vi "pigeon_ver4_1.vi"() -> ()   [LabVIEW 2017]
uses:
  <vilib>/Platform/TimedLoop/XDataNode/timing_clust.ctl
  <vilib>/Platform/TimedLoop/XDataNode/nitl_modes.ctl
  <vilib>/Platform/TimedLoop/XDataNode/wakeup.ctl
  <vilib>/rvi/Emulation/niFpgaGetClockAttributes.vi
  <vilib>/rvi/Emulation/niFpgaSctlEmulationGetInTimedLoop.vi
  <vilib>/rvi/Emulation/niFpgaEmulationReportErrorSimple.vi
  <vilib>/rvi/eio/common/nirviEmuTemplateMethod_errors.vi
  <vilib>/rvi/Emulation/niFpgaProcessEmulError.vi
  <vilib>/rvi/Emulation/niFpgaCriticalErrorInLSC.vi
  <vilib>/rvi/occurrence/nirviWaitOnOccurrenceBase.vi
  <vilib>/rvi/Memory/Memory_Emulation/nirvimemoryFastEmulation.vi
  <vilib>/rvi/Memory/Memory_Emulation/nirvimemoryEmulation.vi
  <vilib>/rvi/Emulation/niFpgaEmulationIsFPGAContextNoSignature.vi
  <vilib>/rvi/DataTransferAndStorage/Container/Common/niFpgaContainerGetUniqueNameForEmu.vi
  <vilib>/rvi/errors/nirviReportUnexpectedCaseInternalError (U32).vi
  <vilib>/rvi/interface/RandomDataEmulation/niFpgaRandomDataHandleErrors.vi
  <vilib>/eio/EIONode/EIONode.xnode
  <vilib>/Platform/TimedLoop/XDataNode/XDataNode.xnode
  <vilib>/rvi/DataTransferAndStorage/Container/XNode/niFpgaContainer.xnode
  <vilib>/rvi/interface/RandomDataEmulation/nirviRandomDataFpgaReadWriteTemplate.vi
  <vilib>/Platform/TimedLoop/XDataNode/XDNodeRunTimeDep.lvlib
panel:
  out "It 2":fxp<+,32,8>
  out "ramp ctr 2":i32
  in  "AO0 2":i16
  out "It":fxp<+,32,8>
  out "ramp ctr":i32
  out "Numeric":i16
  in  "analog ramp on":bool
  out "AI2":i16
  in  "Tab Control":enum32{"pigeon"}(tab)
  in  "Digital Reset":bool
  in  "Emergency Stop":bool
  in  "AO0_pigeon":i16
  in  "AO7":i16
  in  "AO6":i16
  out "trigger AI1":bool
  in  "Tab Control 2":T1(tab)
  out "head ip":u16
  out "nxt ip output":u16
  out "forctr output":u16
  out "curr ip":u16
  out "for ctr":u16
  out "for N":u16
  in  "square wave  on?":bool
  in  "square wave period":i32
  in  "IGBTswitch":bool caption="IGBT Switch circular"
  in  "Manual Override":bool
  in  "circular coil current":i16(slide) scale=0.0..32768.0
  in  "analog ramp period":i16
  in  "analog ramp on  2":bool
  in  "End Current":fxp<+,16,16>
  out "circ coil ramp loop end?":bool=TRUE
  out "ramp start val":fxp<+,15,15>
  out "cooling intensity start val":fxp<+,15,15>
  in  "End Cooling Intensity":fxp<+,16,16>
  in  "cooling intensity ramp on":bool
  out "cooling power ramp loop end?":bool=TRUE
  in  "ramp time [10*us]":fxp<+,16,16>
  out "delta cooling power /dT":fxp<+/-,32,9>
  in  "cooling ramp time [10*us]":fxp<+,16,16>
  out "deltaI/T":fxp<+/-,32,9>
  out "PD1":i16
  out "PD2":i16
  out "PD3":i16
  out "FIFO size":i16
  in  "AO0":i16
  in  "AO1":i16
  in  "AO2":i16
  in  "Run program":bool
  in  "halt processor":bool
  out "control flags":i8 format="%b"
  in  "host operation":i16
  in  "address":u16
  in  "data1":u16
  in  "data2":i32
  in  "repeat program":i32
  out "IP address":i16
  out "PMT1":i16=-4740
  out "ReA":i32
  out "RegB":i16
  out "RegC":i16
  out "exttrigger":bool=TRUE
  out "AI1":i16=161
  out "RegD":i16
  in  "AO4":i16
  in  "AO3":i16
  out "Connector0/AI0":i16
  in  "AO5":i16
  in  "AO5_pigeon":i16
  out "connector 0 DIO":bool[](array[boolean])
  out "connector 1 DIO":bool[](array[boolean])
  out "connector 2 DIO":bool[](array[boolean])
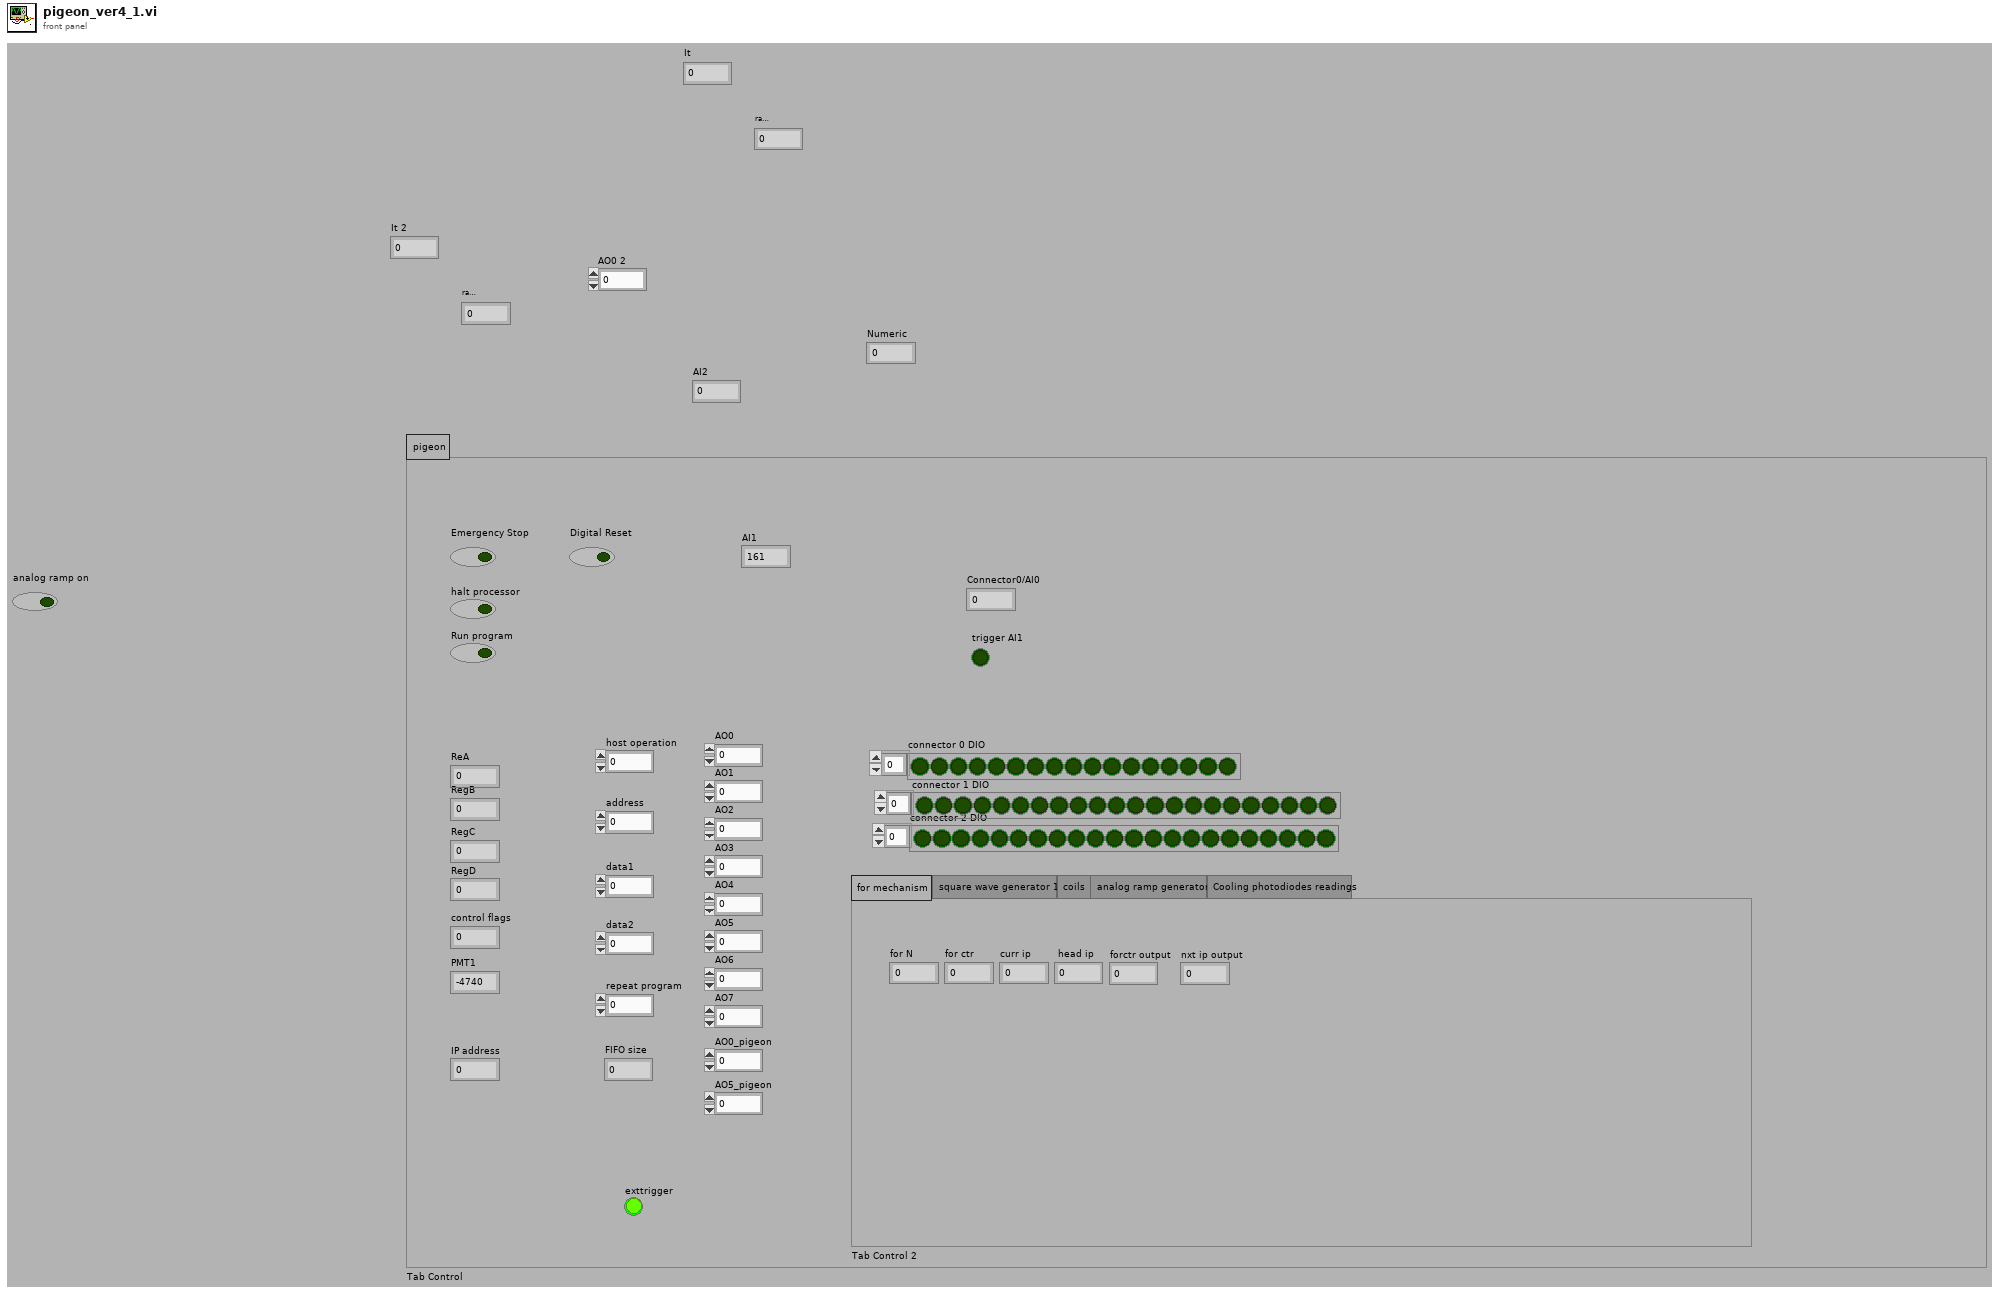
[diagram p1: front panel]
types:
  T1 = enum32{"for mechanism", "square wave generator 1", "coils", "analog ramp generator", "Cooling photodiodes readings"}
  T2 = typedef "XDNodeRunTimeDep.lvlib/timing_clust.ctl" = cluster{"Expected End [f-1]":u64, "Actual End [f-1]":u64, "Finished Late? [f-1]":bool, "Expected End [i-1]":u64, "Actual End [i-1]":u64, "Finished Late? [i-1]":bool, "Expected Start [i]":u64, "Actual Start [i]":u64, "Expected Start [f]":u64, "Actual Start [f]":u64, "Source Name":string, "Structure Name":string, "Period":i64, "Deadline":i64, "Offset":i64, "Start":i64, "Priority":i32, "Timeout":i32, "Mode":T3, "Wakeup Reason":T4, "Error":errorcluster, "Source Type":string, "Secondary Source Type":string, "Global End Time":u64, "Global Start Time":u64, "Frame Duration":u64, "Iteration Duration":u64, "Assigned CPU":i32, "I/O Scan Engine Mode":u32}
  T3 = typedef "XDNodeRunTimeDep.lvlib/nitl_modes.ctl" = enum32{"No Change", "Process missed periods, maintain original phase", "Discard missed periods, maintain original phase", "Process missed periods, ignore original phase", "Discard missed periods, ignore original phase"}
  T4 = typedef "XDNodeRunTimeDep.lvlib/wakeup.ctl" = enum32{"Normal", "Aborted", "Asynchronous wakeup", "Timing source error", "Timed loop error", "Timeout"}
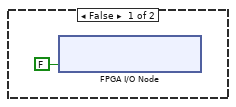
[diagram p2: hidden frame]
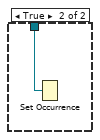
[diagram p3: hidden frame]
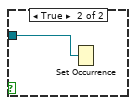
[diagram p5: hidden frame]
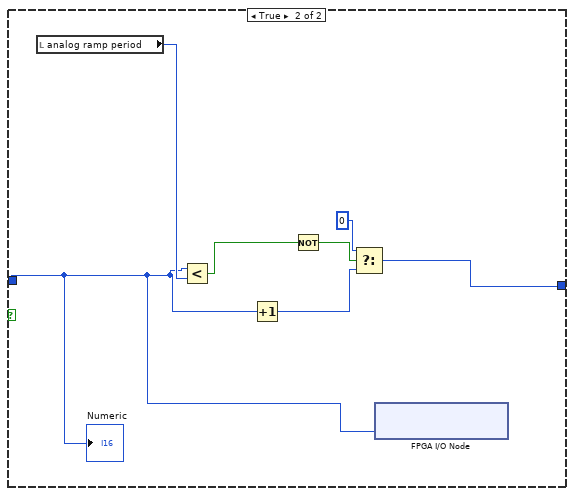
[diagram p6: hidden frame]
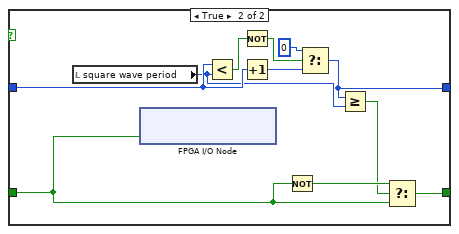
[diagram p7: hidden frame]
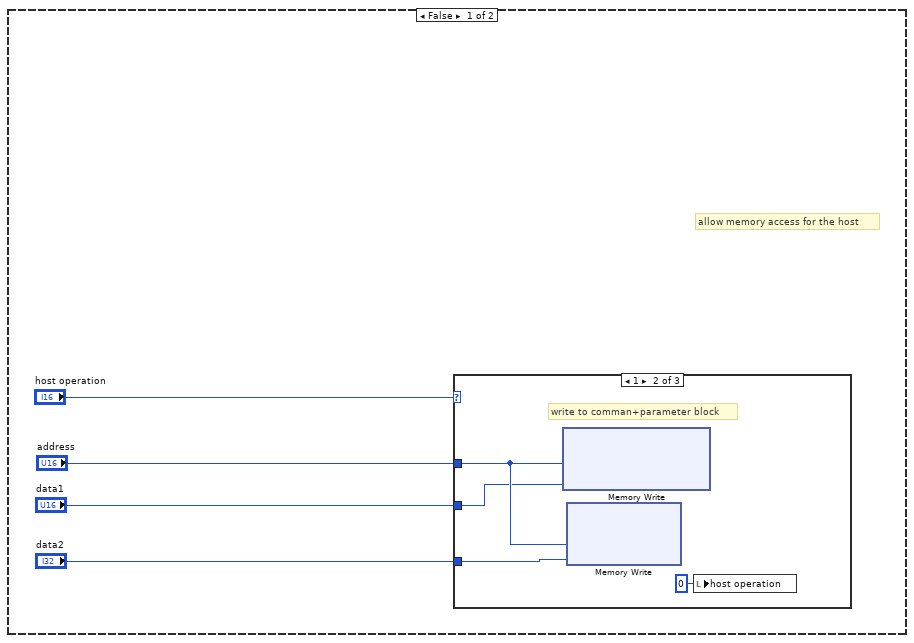
[diagram p8: hidden frame]
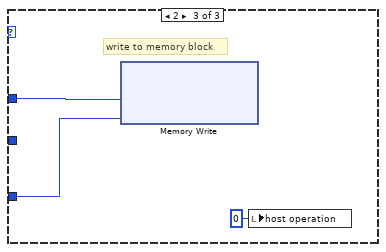
[diagram p10: hidden frame]
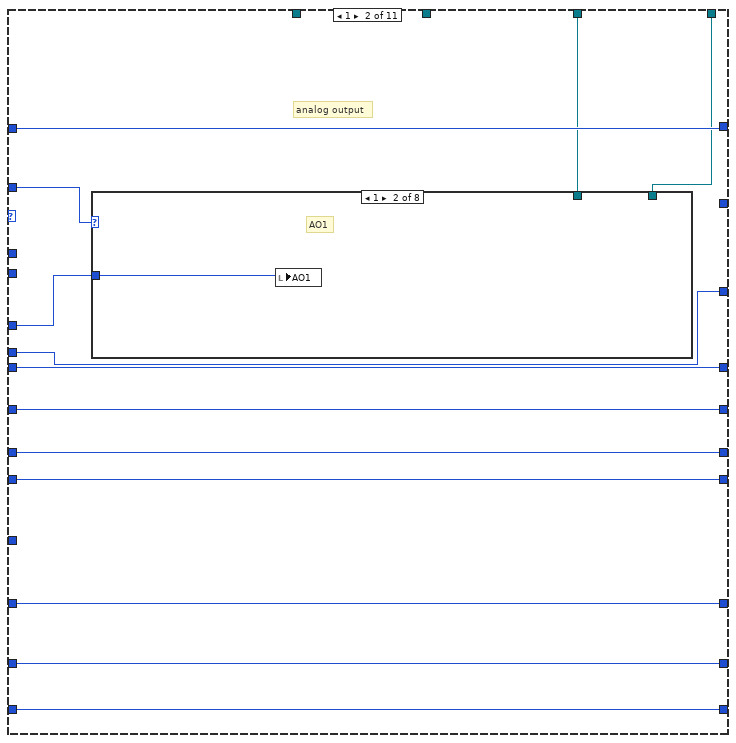
[diagram p12: hidden frame]
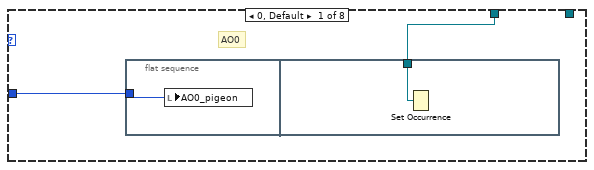
[diagram p13: hidden frame]
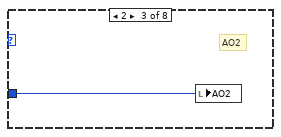
[diagram p14: hidden frame]
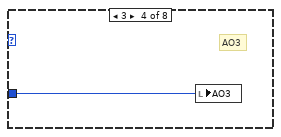
[diagram p15: hidden frame]
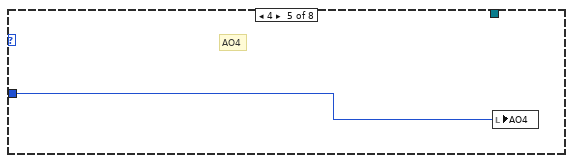
[diagram p16: hidden frame]
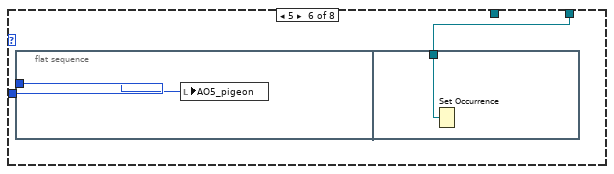
[diagram p17: hidden frame]
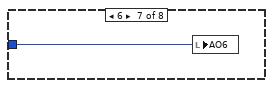
[diagram p18: hidden frame]
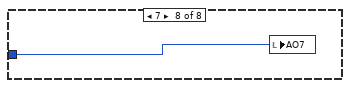
[diagram p19: hidden frame]
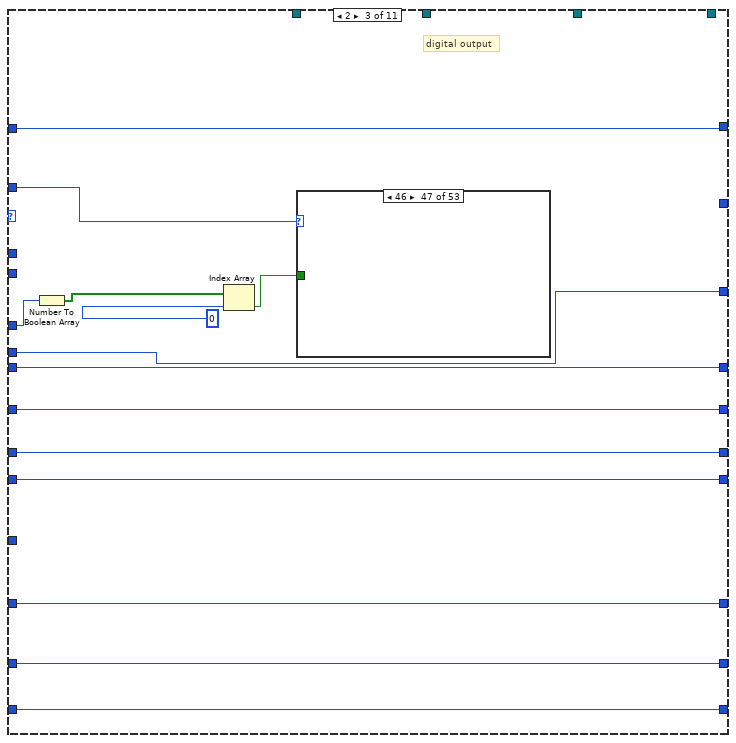
[diagram p20: hidden frame]
diagram:
  w13 = refnum<k21> "40 MHz Onboard Clock" ("FPGA Clock")
  # "circular coil analog ramp occurance"
  # "analog ramp generator"
  # "Analog read block for loading time"
  # "Square Wave Generator Block\nonly Connector1/DIO6 now supports this"
  # "RegB: accumulates flag[0] (results of if condition) to see how many bright events occured\nRegC: loop counter (for GenRepeatSeq)\nRegA: (sub) loop counter (for Gen Wait), #of     photons \nRegB:counter"
  # "flags[0]:result of the if statement\nflags[1]:reset photon counters\nflags[2]:count FIFO size\nflag3[3]:exttrigger\nflag4[4]:trigger MOT fluoresence counter\nflags[7]:halt and exit program"
  # "Digital pin layout\n----------------------------------------------------------------\n\n-----Connector0-----\nC0DIO0-8  -> Rack DIO 0-8\n\n-----Connector2-----\nC2DIO0  -> Rack DI9 external trigger \nC2DIO1-4  -> Rack DIO 10-13\nC2DIO5 -> integrator hold (single BNC)\nC2DIO6-10 D\\A voltage output\nC2DIO22-23 PMTs\nC2DIO32-39 stepmotors control"
  # "analog pin layout\n---------------------------------------------------------------\n\n------connector0-----\nAO0 VCO 422\nAO1 VCO 1092\nAO2 VCO optical pumping\nAO3 408 DC current control\nAO4 422 intensitiy mixer\nAO5 (used to be endcap N) B field feedforward\nAO6 endcap S\nAO7 674 intensity setpoint controller\n\nAI0 B field feed forward"
  n1 = case shown="False" "Digital Reset" {
    frame False {
    }
    frame True {
    }
  }
  n2 = Generate Occurrence() -> (w2:refnum<k4>)
  n3 = while {
    tunnel: w2 -> [w16]
    stop <- FALSE stop-if-true
    n4 = flat-sequence {
      tunnel: w16 -> [w18]
      frame #0 {
        n5 = Wait on Occurrence(2:w18) -> ()  [unwired: 2 in, 1 out]
      }
      frame #1 {
        # "delta I/T"
        n6 = local read "AO5"() -> (w20:i16)
        n7 = To Fixed-Point(number=w20) -> (fixed-point=w19:fxp<+,15,15>)  [unwired: 1 in]
        "cooling intensity start val" <- w19
        n8 = Subtract(x="End Cooling Intensity", y=w19) -> (x-y=w29:fxp<+/-,16,16>)
        n9 = Multiply(x="cooling ramp time [10*us]", y=fxp<+,16,16> 10.0) -> (x*y=w27:fxp<+,32,32>)
        n10 = Divide(x=w29, y=w27) -> (x/y=w28:fxp<+/-,32,16>)
        "delta cooling power /dT" <- w28
        n11 = while {
          tunnel: w28 -> [w41]
          tunnel: w19 -> [w40]
          tunnel: w29 -> [w39]
          tunnel: "End Cooling Intensity" -> [w38]
          shift-right: [w33] -> _
          shift-left: i16 0 -> [w34]
          tunnel: [w31] -> w22
          tunnel: [w30] -> w21
          stop <- w30 stop-if-true
          n12 = flat-sequence {
            tunnel: w38 -> [w44]
            tunnel: w39 -> [w45]
            tunnel: [w45] -> w37
            tunnel: [w44] -> w36
            tunnel: [w43] -> w35
            tunnel: w34 -> [w43]
            tunnel: [w42] -> w32
            tunnel: [w61] -> w30
            tunnel: w41 -> [w60]
            tunnel: w40 -> [w59]
            tunnel: w37 -> [w58]
            tunnel: w36 -> [w57]
            tunnel: w35 -> [w50]
            tunnel: [w51] -> w33
            tunnel: w32 -> [w49]
            tunnel: [w46] -> w31
            frame #0 {
              w42 = u32 2 ("Count(uSec)")
              n13 = call "Loop Timer2"("Count(uSec)"=w42) -> ()  [unwired: 1 out]
            }
            frame #1 {
              # "elapsed time"
              n14 = Multiply(x=w49, y=w50) -> (x*y=w48:fxp<+,15,15>)
              n15 = Increment(x=w50) -> (x+1=w51:i32)
              "ramp ctr 2" <- w51
              n16 = Greater?(x=w58, y=fxp<+/-,31,9> 0.0) -> (0:w54:bool)
              n17 = Multiply(x=w60, y=w48) -> (x*y=w56:fxp<+/-,32,16>)
              n18 = Add(x=w59, y=w56) -> (x+y=w46:fxp<+,15,15>)
              "It 2" <- w46
              n19 = To Word Integer(number=w46) -> (16bit integer=w47:i16)
              n20 = Greater?(x=w46, y=w57) -> (0:w53:bool)
              n21 = Not(x=w53) -> (.not. x?=w52:bool)
              n22 = local write "AO5"(w47) -> ()
              n23 = Select(t=w53, s=w54, f=w52) -> (s? t:f=w61:bool)
            }
          }
        }
        "cooling power ramp loop end?" <- w21
        n24 = local write "cooling intensity start val"(w22) -> ()
      }
    }
  }
  n25 = while {
    tunnel: w2 -> [w63]
    stop <- FALSE stop-if-true
    n26 = case shown="False" "cooling intensity ramp on" {
      tunnel: w63 -> [_ w65]
      frame False {
      }
      frame True {
        n27 = Set Occurrence(w65) -> ()
      }
    }
  }
  n28 = while "Analog out loop" {
    stop <- FALSE stop-if-true
    n29 = Select(t=i16 16385, s="IGBTswitch", f=i16 0) -> (s? t:f=w74:i16)
    n30 = Select(t="circular coil current", s="Manual Override", f="AO0") -> (s? t:f=w68:i16)
    n31 = Select(t=w74, s="Manual Override", f="AO3") -> (s? t:f=w73:i16)
    n32 = xnode "FPGA I/O Node"("Connector0/AO0"=w68, "Connector0/AO1"="AO1", "Connector0/AO2"="AO2", "Connector0/AO3"=w73, "Connector0/AO4"="AO4", "Connector0/AO5"="AO5", "Connector0/AO6"="AO6", "Connector0/AO7"="AO7") -> ("Connector0/AI1"=→"AI1":i16, "Connector0/AI2"=→"AI2":i16)  [unwired: 10 in, 10 out]
  }
  n33 = node-c288(w13) -> (w15:T2)
  n34 = timed-loop {
    timing: w15 -> [_]
    timing-out: [_] -> w14
    shift-right: [w98] -> _
    shift-left: _ -> [w87]
    shift-right: [w91] -> _
    shift-left: _ -> [w100]
    shift-right: [w93] -> _
    shift-left: _ -> [w94]
    stop <- FALSE stop-if-true
    (unwired) FALSE
    n35 = local read "control flags"() -> (w95:i8)
    n36 = xnode "FPGA I/O Node"() -> ("Connector2/DIO0"=→"exttrigger":bool)  [unwired: 1 in, 1 out]
    n37 = xnode "FPGA I/O Node"() -> ("Connector0/DIO0"=w91:bool)  [unwired: 1 in, 1 out]
    n38 = Number To Boolean Array(number=w95) -> (Boolean array=w96:bool[])
    n39 = Increment(x=w87) -> (x+1=w88:u16)
    n40 = Index Array(array=w96, index=1) -> (element=w93:bool)
    n41 = Greater?(x=w91, y=w100) -> (0:w90:bool)
    n42 = Not Equal?(x=w93, y=w94) -> (x != y?=w85:bool)
    n43 = Select(t=w88, s=w90, f=w87) -> (s? t:f=w99:u16)
    n44 = Select(t=u16 0, s=w85, f=w99) -> (s? t:f=w98:u16)
    "PMT1" <- w98
  }
  n45 = Generate Occurrence() -> (w6:refnum<k4>)
  n46 = local write "cooling power ramp loop end?"(FALSE ("ramp loop end?")) -> ()
  n47 = local write "circ coil ramp loop end?"(FALSE ("ramp loop end?")) -> ()
  n48 = node-c288(w14) -> ()
  n49 = while {
    tunnel: w6 -> [w104]
    stop <- FALSE stop-if-true
    n50 = case shown="False" "analog ramp on  2" {
      tunnel: w104 -> [_ w106]
      frame False {
      }
      frame True {
        n51 = Set Occurrence(w106) -> ()
      }
    }
  }
  n52 = while {
    tunnel: w6 -> [w107]
    stop <- FALSE stop-if-true
    n53 = flat-sequence {
      tunnel: w107 -> [w109]
      frame #0 {
        n54 = Wait on Occurrence(2:w109) -> ()  [unwired: 2 in, 1 out]
      }
      frame #1 {
        # "delta I/T"
        n55 = local read "AO0"() -> (w114:i16)
        "ramp start val" <- w114
        n56 = Divide(x=fxp<+,15,15> 220.0, y=i16 32767) -> (x/y=w115:fxp<+,32,16>)
        n57 = Multiply(x=w115, y=w114) -> (x*y=w113:fxp<+/-,48,32>)
        n58 = Subtract(x="End Current", y=w113) -> (x-y=w125:fxp<+/-,32,9>)
        n59 = Multiply(x="ramp time [10*us]", y=fxp<+,16,16> 10.0) -> (x*y=w123:fxp<+,32,32>)
        n60 = Divide(x=w125, y=w123) -> (x/y=w124:fxp<+/-,32,9>)
        "deltaI/T" <- w124
        n61 = Divide(x=fxp<+,15,15> 32767.0, y=fxp<+,6,8> 220.0) -> (x/y=w126:fxp<+,15,15>)
        n62 = while {
          tunnel: w126 -> [w140]
          tunnel: w124 -> [w139]
          tunnel: w113 -> [w138]
          tunnel: w125 -> [w137]
          tunnel: "End Current" -> [w136]
          shift-right: [w130] -> _
          shift-left: i16 0 -> [w131]
          tunnel: [w128] -> w111
          tunnel: [w127] -> w110
          stop <- w127 stop-if-true
          n63 = flat-sequence {
            tunnel: w136 -> [w143]
            tunnel: w137 -> [w144]
            tunnel: w140 -> [w145]
            tunnel: [w145] -> w135
            tunnel: [w144] -> w134
            tunnel: [w143] -> w133
            tunnel: [w142] -> w132
            tunnel: w131 -> [w142]
            tunnel: [w141] -> w129
            tunnel: [w161] -> w127
            tunnel: w139 -> [w160]
            tunnel: w138 -> [w159]
            tunnel: w135 -> [w162]
            tunnel: w134 -> [w158]
            tunnel: w133 -> [w157]
            tunnel: w132 -> [w149]
            tunnel: [w150] -> w130
            tunnel: w129 -> [w148]
            tunnel: [w146] -> w128
            frame #0 {
              w141 = u32 2 ("Count(uSec)")
              n64 = call "Loop Timer"("Count(uSec)"=w141) -> ()  [unwired: 1 out]
            }
            frame #1 {
              # "elapsed time"
              n65 = Multiply(x=w148, y=w149) -> (x*y=w147:u32)
              n66 = Increment(x=w149) -> (x+1=w150:i32)
              "ramp ctr" <- w150
              n67 = Greater?(x=w158, y=fxp<+/-,31,9> 0.0) -> (0:w154:bool)
              n68 = Multiply(x=w160, y=w147) -> (x*y=w156:fxp<+/-,32,9>)
              n69 = Add(x=w159, y=w156) -> (x+y=w153:fxp<+,32,8>)
              "It" <- w153
              n70 = Multiply(x=w162, y=w153) -> (x*y=w146:i16)
              n71 = Greater?(x=w153, y=w157) -> (0:w152:bool)
              n72 = local write "AO0"(w146) -> ()
              n73 = Not(x=w152) -> (.not. x?=w151:bool)
              n74 = Select(t=w152, s=w154, f=w151) -> (s? t:f=w161:bool)
            }
          }
        }
        "circ coil ramp loop end?" <- w110
        n75 = local write "ramp start val"(w111) -> ()
      }
    }
  }
  n76 = while {
    shift-right: [w163] -> _
    shift-left: _ -> [w165]
    stop <- FALSE stop-if-true
    # "write Pulse to conn2/Dio26 on low->high transition of dio12. used for the trigger channel (channel 3) of the time tagger"
    n77 = xnode "FPGA I/O Node"() -> ("Connector2/DIO12"=w166:bool)  [unwired: 1 in, 1 out]
    n78 = Not(x=w165) -> (.not. x?=w164:bool)
    n79 = feedback-in #1(w166) -> ()
    n80 = feedback #1() -> (w163:bool)  [unwired: 1 in]
    n81 = case shown="True" w163 {
      frame False {
        n82 = xnode "FPGA I/O Node"("Connector2/DIO26"=FALSE) -> ()  [unwired: 1 in, 1 out]
      }
      frame True {
        n83 = call "Wait"("Count(uSec)"=u32 1) -> ()  [unwired: 1 out]
        n84 = xnode "FPGA I/O Node"("Connector2/DIO26"=TRUE) -> ()  [unwired: 1 in, 1 out]
      }
    }
    n85 = And(x=w164, y=w163) -> ()  [unwired: 1 out]
  }
  n86 = while {
    stop <- FALSE stop-if-true
    n87 = xnode "FPGA I/O Node"() -> ("Connector0/AI1"=→"PD1":i16, "Connector0/AI2"=→"PD2":i16, "Connector0/AI3"=→"PD3":i16)  [unwired: 3 in, 3 out]
  }
  n88 = Generate Occurrence() -> (w5:refnum<k4>)
  n89 = while {
    tunnel: w5 -> [w176]
    stop <- FALSE stop-if-true
    n90 = flat-sequence {
      tunnel: w176 -> [w177]
      frame #0 {
        n91 = Wait on Occurrence(2:w177) -> ()  [unwired: 2 in, 1 out]
      }
      frame #1 {
        n92 = local read "AO0_pigeon"() -> (w178:i16)
        n93 = local write "AO0"(w178) -> ()
      }
    }
  }
  n94 = while {
    stop <- FALSE stop-if-true
    n95 = xnode "FPGA I/O Node"() -> ("Connector0/DIO0"=w241:bool, "Connector0/DIO1"=w240:bool, "Connector0/DIO2"=w239:bool, "Connector0/DIO3"=w238:bool, "Connector0/DIO4"=w237:bool, "Connector0/DIO5"=w236:bool, "Connector0/DIO6"=w235:bool, "Connector0/DIO7"=w234:bool, "Connector0/DIO8"=w233:bool, "Connector0/DIO9"=w232:bool, "Connector0/DIO10"=w231:bool, "Connector0/DIO11"=w230:bool, "Connector0/DIO12"=w229:bool, "Connector0/DIO13"=w228:bool, "Connector0/DIO14"=w227:bool, "Connector0/DIO15"=w226:bool)  [unwired: 16 in, 16 out]
    n96 = Build Array(w241, w240, w239, w238, w238, w237, w236, w235, w234, w233, w232, w231, w230, w229, w228, w227, w226) -> (→"connector 0 DIO":bool[])
    n97 = xnode "FPGA I/O Node"() -> ("Connector1/DIO0"=w224:bool, "Connector1/DIO1"=w223:bool, "Connector1/DIO2"=w222:bool, "Connector1/DIO3"=w221:bool, "Connector1/DIO4"=w220:bool, "Connector1/DIO5"=w219:bool, "Connector1/DIO6"=w218:bool, "Connector1/DIO7"=w217:bool, "Connector1/DIO8"=w216:bool, "Connector1/DIO9"=w215:bool, "Connector1/DIO10"=w214:bool, "Connector1/DIO11"=w213:bool, "Connector1/DIO12"=w212:bool, "Connector1/DIO13"=w211:bool, "Connector1/DIO15"=w210:bool, "Connector1/DIO16"=w209:bool, "Connector1/DIO17"=w208:bool, "Connector1/DIO18"=w207:bool, "Connector1/DIO19"=w206:bool, "Connector1/DIO20"=w205:bool, "Connector1/DIO21"=w204:bool, "Connector1/DIO22"=w203:bool)  [unwired: 23 in, 24 out]
    n98 = Build Array(w224, w223, w222, w221, w220, w219, w218, w217, w216, w215, w214, w213, w212, w211, w210, w209, w208, w207, w206, w205, w204, w203) -> (→"connector 1 DIO":bool[])
    n99 = xnode "FPGA I/O Node"() -> ("Connector2/DIO0"=w201:bool, "Connector2/DIO1"=w200:bool, "Connector2/DIO2"=w199:bool, "Connector2/DIO3"=w198:bool, "Connector2/DIO4"=w197:bool, "Connector2/DIO5"=w196:bool, "Connector2/DIO6"=w195:bool, "Connector2/DIO7"=w194:bool, "Connector2/DIO8"=w193:bool, "Connector2/DIO9"=w192:bool, "Connector2/DIO10"=w191:bool, "Connector2/DIO11"=w190:bool, "Connector2/DIO12"=w189:bool, "Connector2/DIO12"=w188:bool, "Connector2/DIO14"=w187:bool, "Connector2/DIO15"=w186:bool, "Connector2/DIO16"=w185:bool, "Connector2/DIO17"=w184:bool, "Connector2/DIO18"=w183:bool, "Connector2/DIO19"=w182:bool, "Connector2/DIO20"=w181:bool, "Connector2/DIO21"=w180:bool)  [unwired: 23 in, 24 out]
    n100 = Build Array(w201, w200, w199, w198, w197, w196, w195, w194, w193, w192, w191, w190, w189, w188, w187, w186, w185, w184, w183, w182, w181, w180) -> (→"connector 2 DIO":bool[])
  }
  n101 = Generate Occurrence() -> (w3:refnum<k4>)
  n102 = while "main loop" {
    tunnel: w13 -> [w247]
    tunnel: w6 -> [w246]
    tunnel: w5 -> [w245]
    tunnel: w3 -> [w244]
    tunnel: w2 -> [w243]
    stop <- FALSE ("stop") stop-if-true
    n103 = case shown="True" "Run program" {
      tunnel: w247 -> [_ w265]
      tunnel: w246 -> [_ w264]
      tunnel: w245 -> [_ w263]
      tunnel: w244 -> [_ w262]
      tunnel: w243 -> [_ w261]
      frame False {
        # "allow memory access for the host"
        n104 = case shown="1" "host operation" {
          tunnel: "address" -> [_ w255 w260]
          tunnel: "data1" -> [_ w254 _]
          tunnel: "data2" -> [_ w257 w258]
          frame 0, Default {
          }
          frame 1 {
            # "write to comman+parameter block"
            n105 = xnode ("Memory Write")("Address"=w255, "Data"=w254) -> ()  [unwired: 1 in, 1 out]
            n106 = xnode ("Memory Write")("Address"=w255, "Data"=w257) -> ()  [unwired: 1 in, 1 out]
            n107 = local write "host operation"(i16 0 ("host operation")) -> ()
          }
          frame 2 {
            # "write to memory block"
            n108 = xnode ("Memory Write")("Address"=w260, "Data"=w258) -> ()  [unwired: 1 in, 1 out]
            n109 = local write "host operation"(i16 0 ("host operation")) -> ()
          }
        }
      }
      frame True {
        n110 = flat-sequence {
          tunnel: w265 -> [w271]
          tunnel: w264 -> [w269]
          tunnel: w263 -> [w268]
          tunnel: w262 -> [w267]
          tunnel: w261 -> [w266]
          frame #0 {
            n111 = for {
              N: "repeat program" -> [_]
              tunnel: w271 -> [w280]
              shift-right: [w278] -> _
              shift-left: i16 0 -> [w279]
              tunnel: w269 -> [w277]
              tunnel: w268 -> [w276]
              tunnel: w267 -> [w274]
              tunnel: w266 -> [w273]
              n112 = case shown="False" "Emergency Stop" {
                tunnel: w280 -> [w297 _]
                tunnel: w279 -> [w289 w865]
                tunnel: [w288 w865] -> w278
                tunnel: w277 -> [w286 _]
                tunnel: w276 -> [w285 _]
                tunnel: w274 -> [w284 _]
                tunnel: w273 -> [w283 _]
                frame False {
                  # "for head ip (int16)"
                  # "for cntr (int16)"
                  # "ctrl flags"
                  # "Sleep ctr"
                  # "RegD"
                  # "RegD"
                  # "Sleep counter"
                  # "flags"
                  # "RegC"
                  # "RegB"
                  # "RegA"
                  # "RegC"
                  # "RegB"
                  # "RegA (int32)"
                  # "IP"
                  # "IP"
                  n113 = local read "control flags"() -> (w292:i8)
                  n114 = Number To Boolean Array(number=w292) -> (Boolean array=w296:bool[])
                  n115 = node-c288(w297) -> (w303:T2)
                  n116 = Replace Array Subset(array=w296, new element=FALSE ("new element/subarray"), index=7) -> (w294:bool[])
                  n117 = Boolean Array To Number(Boolean array=w294) -> (number=w295:u8)
                  n118 = timed-loop {
                    timing: w303 -> [_]
                    timing-out: [_] -> w302
                    shift-right: [w347] -> _
                    shift-left: i16 0 -> [w305]
                    shift-right: [w343] -> _
                    shift-left: 0 -> [w339]
                    shift-right: [w355] -> _
                    shift-left: i16 0 -> [w346]
                    shift-right: [w354] -> _
                    shift-left: i16 0 -> [w338]
                    shift-right: [w344] -> _
                    shift-left: w295 -> [w345]
                    shift-right: [w337] -> _
                    shift-left: i16 0 -> [w329]
                    shift-right: [w320] -> w288
                    shift-left: w289 -> [w319]
                    shift-right: [w317] -> _
                    shift-left: i16 0 -> [w318]
                    tunnel: w286 -> [w313]
                    tunnel: w285 -> [w312]
                    tunnel: w284 -> [w311]
                    tunnel: w283 -> [w310]
                    shift-right: [w308] -> _
                    shift-left: u16 1 -> [w309]
                    shift-right: [w307] -> _
                    shift-left: i16 0 -> [w306]
                    stop <- w350 stop-if-true
                    # "RegD"
                    # "IP"
                    # "RegC"
                    # "RegB"
                    # "RegA"
                    # "par1"
                    # "par2"
                    # "subcommand"
                    # "command"
                    n119 = xnode ("Memory Read")("Address"=w338) -> ("Data"=w342:i16)  [unwired: 2 in, 2 out]
                    n120 = xnode ("Memory Read")("Address"=w305) -> ("Data"=w326:u16)  [unwired: 1 in, 1 out]
                    n121 = xnode ("Memory Read")("Address"=w305) -> ("Data"=w322:i32)  [unwired: 1 in, 1 out]
                    n122 = Greater Than 0?(x=w329) -> (x > 0?=w324:bool)
                    n123 = Decrement(x=w329) -> (x-1=w330:u32)
                    n124 = Less?(x=w329, y=u32 2) -> (x < y?=w328:bool)
                    n125 = Select(t=w330, s=w324, f=w329) -> (s? t:f=w327:u32)
                    n126 = feedback-in #2(w322) -> ()
                    n127 = feedback #2(u32 0 ("Data")) -> (w321:u32)
                    n128 = feedback-in #3(w342) -> ()
                    n129 = feedback #3(0) -> (w341:i32)
                    n130 = feedback-in #4(w326) -> ()
                    n131 = feedback #4(u16 0 ("Data")) -> (w323:u16)
                    n132 = Increment(x=w305) -> (x+1=w331:u16)
                    n133 = Select(t=0, s=w324, f=w321) -> (s? t:f=w334:u32)
                    n134 = Select(t=w331, s=w328, f=w305) -> (s? t:f=w336:u16)
                    n135 = Select(t=u16 0, s=w324, f=w323) -> (s? t:f=w335:u16)
                    n136 = Split Number(x=w335) -> (hi(x)=w356:u8, lo(x)=w304:u8)
                    n137 = Split Number(x=w334) -> (hi(x)=w348:u16, lo(x)=w349:u16)
                    n138 = case shown="4" w304 {
                      tunnel: w349 -> [_ w378 w399 _ w508 w672 w747 _ _ w811 _]
                      tunnel: w348 -> [_ _ _ _ w501 w671 w746 _ _ w812 _]
                      tunnel: w356 -> [_ w379 w407 w471 w509 w676 _ w766 _ w793 _]
                      tunnel: w339 -> [w366 w377 w406 w463 w507 w673 w751 w770 w787 w810 w852]
                      tunnel: [w366 w377 w406 w463 w504 w673 w751 w770 w787 w809 w852] -> w343
                      tunnel: w346 -> [w365 w376 w405 w462 w506 w674 w752 w769 w790 w808 w853]
                      tunnel: w338 -> [w364 w375 w404 w469 w505 w675 w753 w768 w789 w806 w854]
                      tunnel: [w365 w376 w405 w461 w503 w674 w752 w769 w790 w807 w853] -> w355
                      tunnel: [w364 w375 w404 w469 w502 w675 w753 w768 w789 w805 w854] -> w354
                      tunnel: [w362 w374 w403 w470 w497 w679 w745 w772 w788 w795 w851] -> w347
                      tunnel: w336 -> [w362 w374 w403 w470 w498 w679 _ w772 w788 w796 w851]
                      tunnel: [w363 w373 w402 w467 w499 w678 w744 w761 w784 w799 w857] -> w344
                      tunnel: w345 -> [w363 w373 w402 w468 w500 w677 w744 w760 w783 w800 w857]
                      tunnel: w341 -> [_ _ _ _ w491 w670 _ _ _ _ _]
                      tunnel: w327 -> [w361 w372 w397 w466 w496 w669 w743 w758 w780 w802 w858]
                      tunnel: [w361 w372 w397 w466 w495 w669 w743 w758 w780 w801 w858] -> w337
                      tunnel: w319 -> [w360 w371 w396 w465 w494 w668 w742 w757 w779 w797 w856]
                      tunnel: [w360 w371 w396 w465 w494 w668 w742 w756 w779 w798 w856] -> w320
                      tunnel: w318 -> [w359 w370 w395 w464 w493 w667 w741 w755 w778 w804 w855]
                      tunnel: [w359 w370 w395 w464 w492 w667 w741 w755 w778 w803 w855] -> w317
                      tunnel: w313 -> [_ _ _ _ _ _ _ _ _ w794 _]
                      tunnel: w312 -> [_ w369 _ _ _ _ _ _ _ _ _]
                      tunnel: w311 -> [_ w368 _ _ _ _ _ _ _ _ _]
                      tunnel: w310 -> [_ _ _ _ _ _ _ _ _ w792 _]
                      tunnel: w309 -> [w358 w367 w394 w460 w490 w666 w740 w754 w777 w791 w849]
                      tunnel: [w358 w367 w394 w460 w489 w666 w740 w754 w777 w791 w849] -> w308
                      tunnel: w306 -> [w357 _ _ _ w488 _ _ _ _ _ _]
                      tunnel: [w357 _ _ _ w487 _ _ _ _ _ _] -> w307
                      frame 0, Default {
                      }
                      frame 1 {
                        # "analog output"
                        n139 = case shown="1" w379 {
                          tunnel: w378 -> [w381 w384 w385 w386 w387 w389 w392 w393]
                          tunnel: w369 -> [w380 _ _ _ _ _ _ _]
                          tunnel: w368 -> [_ _ _ _ _ w388 _ _]
                          frame 0, Default {
                            # "AO0"
                            n140 = flat-sequence {
                              tunnel: w381 -> [w382]
                              tunnel: w380 -> [w383]
                              frame #0 {
                                n141 = local write "AO0_pigeon"(w382) -> ()
                              }
                              frame #1 {
                                n142 = Set Occurrence(w383) -> ()
                              }
                            }
                          }
                          frame 1 {
                            # "AO1"
                            n143 = local write "AO1"(w384) -> ()
                          }
                          frame 2 {
                            # "AO2"
                            n144 = local write "AO2"(w385) -> ()
                          }
                          frame 3 {
                            # "AO3"
                            n145 = local write "AO3"(w386) -> ()
                          }
                          frame 4 {
                            # "AO4"
                            n146 = local write "AO4"(w387) -> ()
                          }
                          frame 5 {
                            n147 = flat-sequence {
                              tunnel: w389 -> [w390]
                              tunnel: w388 -> [w391]
                              frame #0 {
                                n148 = local write "AO5_pigeon"(w390) -> ()
                              }
                              frame #1 {
                                n149 = Set Occurrence(w391) -> ()
                              }
                            }
                          }
                          frame 6 {
                            n150 = local write "AO6"(w392) -> ()
                          }
                          frame 7 {
                            n151 = local write "AO7"(w393) -> ()
                          }
                        }
                      }
                      frame 2 {
                        # "digital output"
                        n152 = Number To Boolean Array(number=w399) -> (Boolean array=w400:bool[])
                        n153 = Index Array(array=w400, index=0) -> (element=w398:bool)
                        n154 = case shown="46" w407 {
                          tunnel: w398 -> [w408 w409 w410 w411 w412 w413 w414 w415 w416 w417 w418 w419 w420 w421 w422 w423 w424 w425 w426 w427 w428 w429 w430 w431 w432 w433 w434 w435 w436 w437 w438 w439 w440 w441 w442 w443 w444 w445 w446 w447 w448 w449 w450 w451 w452 w453 _ w454 w455 w456 w457 w458 w459]
                          frame 0, Default {
                            # "write single bit  to DIOPORT0"
                            n155 = xnode "FPGA I/O Node"("Connector1/DIO0"=w408) -> ()  [unwired: 1 in, 1 out]
                          }
                          frame 1 {
                            # "write single bit  to DIOPORT0"
                            n156 = xnode "FPGA I/O Node"("Connector1/DIO1"=w409) -> ()  [unwired: 1 in, 1 out]
                          }
                          frame 2 {
                            # "write single bit  to DIOPORT0"
                            n157 = xnode "FPGA I/O Node"("Connector1/DIO2"=w410) -> ()  [unwired: 1 in, 1 out]
                          }
                          frame 3 {
                            # "write single bit  to DIOPORT0"
                            n158 = xnode "FPGA I/O Node"("Connector1/DIO3"=w411) -> ()  [unwired: 1 in, 1 out]
                          }
                          frame 4 {
                            # "write single bit  to DIOPORT0"
                            n159 = xnode "FPGA I/O Node"("Connector1/DIO4"=w412) -> ()  [unwired: 1 in, 1 out]
                          }
                          frame 5 {
                            # "write single bit  to DIOPORT0"
                            n160 = xnode "FPGA I/O Node"("Connector1/DIO5"=w413) -> ()  [unwired: 1 in, 1 out]
                          }
                          frame 6 {
                            # "write single bit  to DIOPORT0"
                            n161 = xnode "FPGA I/O Node"("Connector1/DIO6"=w414) -> ()  [unwired: 1 in, 1 out]
                          }
                          frame 7 {
                            # "write single bit  to DIOPORT0"
                            n162 = xnode "FPGA I/O Node"("Connector1/DIO7"=w415) -> ()  [unwired: 1 in, 1 out]
                          }
                          frame 8 {
                            # "write single bit  to DIOPORT0"
                            n163 = xnode "FPGA I/O Node"("Connector1/DIO8"=w416) -> ()  [unwired: 1 in, 1 out]
                          }
                          frame 9 {
                            n164 = xnode "FPGA I/O Node"("Connector1/DIO9"=w417) -> ()  [unwired: 1 in, 1 out]
                          }
                          frame 10 {
                            n165 = xnode "FPGA I/O Node"("Connector1/DIO10"=w418) -> ()  [unwired: 1 in, 1 out]
                          }
                          frame 11 {
                            n166 = xnode "FPGA I/O Node"("Connector1/DIO11"=w419) -> ()  [unwired: 1 in, 1 out]
                          }
                          frame 12 {
                            n167 = xnode "FPGA I/O Node"("Connector1/DIO12"=w420) -> ()  [unwired: 1 in, 1 out]
                          }
                          frame 13 {
                            n168 = xnode "FPGA I/O Node"("Connector1/DIO13"=w421) -> ()  [unwired: 1 in, 1 out]
                          }
                          frame 14 {
                            n169 = xnode "FPGA I/O Node"("Connector1/DIO14"=w422) -> ()  [unwired: 1 in, 1 out]
                          }
                          frame 15 {
                            n170 = xnode "FPGA I/O Node"("Connector1/DIO15"=w423) -> ()  [unwired: 1 in, 1 out]
                          }
                          frame 16 {
                            n171 = xnode "FPGA I/O Node"("Connector1/DIO16"=w424) -> ()  [unwired: 1 in, 1 out]
                          }
                          frame 17 {
                            n172 = xnode "FPGA I/O Node"("Connector1/DIO17"=w425) -> ()  [unwired: 1 in, 1 out]
                          }
                          frame 18 {
                            n173 = xnode "FPGA I/O Node"("Connector1/DIO18"=w426) -> ()  [unwired: 1 in, 1 out]
                          }
                          frame 19 {
                            n174 = xnode "FPGA I/O Node"("Connector1/DIO19"=w427) -> ()  [unwired: 1 in, 1 out]
                          }
                          frame 20 {
                            n175 = xnode "FPGA I/O Node"("Connector2/DIO0"=w428) -> ()  [unwired: 1 in, 1 out]
                          }
                          frame 21 {
                            n176 = xnode "FPGA I/O Node"("Connector2/DIO1"=w429) -> ()  [unwired: 1 in, 1 out]
                          }
                          frame 22 {
                            n177 = xnode "FPGA I/O Node"("Connector2/DIO2"=w430) -> ()  [unwired: 1 in, 1 out]
                          }
                          frame 23 {
                            n178 = xnode "FPGA I/O Node"("Connector2/DIO3"=w431) -> ()  [unwired: 1 in, 1 out]
                          }
                          frame 24 {
                            n179 = xnode "FPGA I/O Node"("Connector2/DIO4"=w432) -> ()  [unwired: 1 in, 1 out]
                          }
                          frame 25 {
                            n180 = xnode "FPGA I/O Node"("Connector2/DIO5"=w433) -> ()  [unwired: 1 in, 1 out]
                          }
                          frame 26 {
                            n181 = xnode "FPGA I/O Node"("Connector2/DIO6"=w434) -> ()  [unwired: 1 in, 1 out]
                          }
                          frame 27 {
                            n182 = xnode "FPGA I/O Node"("Connector2/DIO7"=w435) -> ()  [unwired: 1 in, 1 out]
                          }
                          frame 28 {
                            n183 = xnode "FPGA I/O Node"("Connector2/DIO8"=w436) -> ()  [unwired: 1 in, 1 out]
                          }
                          frame 29 {
                            n184 = xnode "FPGA I/O Node"("Connector2/DIO9"=w437) -> ()  [unwired: 1 in, 1 out]
                          }
                          frame 30 {
                            n185 = xnode "FPGA I/O Node"("Connector2/DIO10"=w438) -> ()  [unwired: 1 in, 1 out]
                          }
                          frame 31 {
                            n186 = xnode "FPGA I/O Node"("Connector2/DIO11"=w439) -> ()  [unwired: 1 in, 1 out]
                          }
                          frame 32 {
                            n187 = xnode "FPGA I/O Node"("Connector2/DIO12"=w440) -> ()  [unwired: 1 in, 1 out]
                          }
                          frame 33 {
                            n188 = xnode "FPGA I/O Node"("Connector2/DIO13"=w441) -> ()  [unwired: 1 in, 1 out]
                          }
                          frame 34 {
                            n189 = xnode "FPGA I/O Node"("Connector2/DIO14"=w442) -> ()  [unwired: 1 in, 1 out]
                          }
                          frame 35 {
                            n190 = xnode "FPGA I/O Node"("Connector2/DIO15"=w443) -> ()  [unwired: 1 in, 1 out]
                          }
                          frame 36 {
                            n191 = xnode "FPGA I/O Node"("Connector2/DIO16"=w444) -> ()  [unwired: 1 in, 1 out]
                          }
                          frame 37 {
                            n192 = xnode "FPGA I/O Node"("Connector2/DIO17"=w445) -> ()  [unwired: 1 in, 1 out]
                          }
                          frame 38 {
                            n193 = xnode "FPGA I/O Node"("Connector2/DIO18"=w446) -> ()  [unwired: 1 in, 1 out]
                          }
                          frame 39 {
                            n194 = xnode "FPGA I/O Node"("Connector2/DIO19"=w447) -> ()  [unwired: 1 in, 1 out]
                          }
                          frame 40 {
                            n195 = xnode "FPGA I/O Node"("Connector2/DIO20"=w448) -> ()  [unwired: 1 in, 1 out]
                          }
                          frame 41 {
                            n196 = xnode "FPGA I/O Node"("Connector2/DIO21"=w449) -> ()  [unwired: 1 in, 1 out]
                          }
                          frame 42 {
                            n197 = xnode "FPGA I/O Node"("Connector2/DIO22"=w450) -> ()  [unwired: 1 in, 1 out]
                          }
                          frame 43 {
                            n198 = xnode "FPGA I/O Node"("Connector2/DIO23"=w451) -> ()  [unwired: 1 in, 1 out]
                          }
                          frame 44 {
                            n199 = xnode "FPGA I/O Node"("Connector2/DIO24"=w452) -> ()  [unwired: 1 in, 1 out]
                          }
                          frame 45 {
                            n200 = xnode "FPGA I/O Node"("Connector2/DIO25"=w453) -> ()  [unwired: 1 in, 1 out]
                          }
                          frame 46 {
                          }
                          frame 47 {
                            n201 = xnode "FPGA I/O Node"("Connector2/DIO27"=w454) -> ()  [unwired: 1 in, 1 out]
                          }
                          frame 48 {
                            n202 = xnode "FPGA I/O Node"("Connector2/DIO28"=w455) -> ()  [unwired: 1 in, 1 out]
                          }
                          frame 49 {
                            n203 = xnode "FPGA I/O Node"("Connector2/DIO29"=w456) -> ()  [unwired: 1 in, 1 out]
                          }
                          frame 50 {
                            n204 = xnode "FPGA I/O Node"("Connector2/DIO30"=w457) -> ()  [unwired: 1 in, 1 out]
                          }
                          frame 51 {
                            n205 = xnode "FPGA I/O Node"("Connector2/DIO31"=w458) -> ()  [unwired: 1 in, 1 out]
                          }
                          frame 52 {
                            n206 = xnode "FPGA I/O Node"("Connector2/DIO32"=w459) -> ()  [unwired: 1 in, 1 out]
                          }
                        }
                      }
                      frame 3 {
                        # "photon counting"
                        n207 = case shown="3" w471 {
                          tunnel: [w472 w474 w486] -> w461
                          tunnel: w462 -> [w472 w475 w486]
                          tunnel: w468 -> [w473 w477 w484]
                          tunnel: [w473 w477 w483] -> w467
                          frame 2, Default {
                          }
                          frame 1 {
                            # "PMT1"
                            n208 = local read "PMT1"() -> (w476:i16)
                            n209 = Add(x=w476, y=w475) -> (x+y=w474:u16)
                          }
                          frame 3 {
                            # "Reset  photon counter"
                            # "make a Not gate of flag(1)"
                            n210 = Number To Boolean Array(number=w484) -> (Boolean array=w481:bool[])
                            n211 = Index Array(array=w481, index=1) -> (element=w479:bool)
                            n212 = Not(x=w479) -> (.not. x?=w478:bool)
                            n213 = Replace Array Subset(array=w481, new element=w478, index=1) -> (w482:bool[])
                            n214 = Boolean Array To Number(Boolean array=w482) -> (number=w483:u8)
                          }
                        }
                      }
                      frame 4 {
                        # "registers operation"
                        n215 = case shown="13" w509 {
                          tunnel: w508 -> [w517 w529 w538 _ _ _ _ w590 _ w610 w625 _ _ w656]
                          tunnel: w507 -> [_ w528 w537 w546 w556 w566 w572 w595 w603 w615 w630 w646 w653 _]
                          tunnel: w506 -> [w520 _ w536 w545 w558 w565 w580 w594 w599 w613 w628 w645 w652 _]
                          tunnel: w505 -> [w519 w527 _ w548 w557 _ w573 w593 w602 w614 w629 w644 w651 _]
                          tunnel: [w516 w528 w537 w546 w555 w566 w572 w595 w603 w615 w630 w646 w653 _] -> w504
                          tunnel: [w520 w529 w536 w545 w558 w565 w579 w594 w601 w613 w628 w645 w652 _] -> w503
                          tunnel: [w519 w527 w538 w547 w557 w565 w573 w593 w602 w614 w629 w644 w651 _] -> w502
                          tunnel: w501 -> [w518 _ _ _ _ _ _ w591 _ _ w624 _ _ w657]
                          tunnel: w500 -> [w515 w526 w535 w544 w554 w564 w574 w592 w606 w618 w633 w643 w648 _]
                          tunnel: [w515 w526 w535 w544 w554 w564 w574 w592 w606 w618 w633 w643 w648 _] -> w499
                          tunnel: w498 -> [w514 w525 w534 w543 w553 w563 w571 w584 w605 w617 w632 w638 w647 w659]
                          tunnel: [w514 w525 w534 w543 w553 w563 w571 w587 w605 w617 w632 w641 w647 w665] -> w497
                          tunnel: w496 -> [w513 w524 w533 w542 w552 w562 w570 _ w604 w616 w631 _ w649 _]
                          tunnel: [w513 w524 w533 w542 w552 w562 w570 w588 w604 w616 w631 w636 w649 _] -> w495
                          tunnel: w493 -> [w512 w523 w532 w541 w551 w561 w569 w583 w598 _ w623 w637 w650 _]
                          tunnel: [w512 w523 w532 w541 w551 w561 w569 w583 w598 w611 w622 w637 w650 _] -> w492
                          tunnel: w491 -> [_ _ _ _ _ _ _ _ _ _ _ w636 _ _]
                          tunnel: w490 -> [w511 w522 w531 w540 w550 w560 w568 w582 w597 w608 w620 w635 _ w664]
                          tunnel: [w511 w522 w531 w540 w550 w560 w568 w582 w597 w608 w620 w635 u16 1 w663] -> w489
                          tunnel: w488 -> [w510 w521 w530 w539 w549 w559 w567 w581 w596 w607 w619 w634 _ _]
                          tunnel: [w510 w521 w530 w539 w549 w559 w567 w581 w596 w607 w619 w634 w647 w658] -> w487
                          frame 0, Default {
                            # "Set par1,2 to RegA"
                            n216 = Join Numbers(hi=w518, lo=w517) -> ((hi.lo)=w516:u32)
                          }
                          frame 1 {
                            # "Set par1 to RegB"
                          }
                          frame 2 {
                            # "Set par1 to RegC"
                          }
                          frame 3 {
                            # "increase RegC by 1"
                            n217 = Increment(x=w548) -> (x+1=w547:u16)
                          }
                          frame 4 {
                            # "increase RegA by 1"
                            n218 = Increment(x=w556) -> (x+1=w555:u32)
                          }
                          frame 5 {
                            # "Set regC to regB"
                          }
                          frame 6 {
                            # "regB<-regB+flags[0]"
                            n219 = Number To Boolean Array(number=w574) -> (Boolean array=w578:bool[])
                            n220 = Index Array(array=w578, index=0) -> (element=w576:bool)
                            n221 = Boolean To (0,1)(Boolean=w576) -> (0, 1=w575:i16)
                            n222 = Add(x=w575, y=w580) -> (x+y=w579:u16)
                          }
                          frame 7 {
                            # "Sleep counter = [par1 par2]"
                            n223 = Join Numbers(hi=w591, lo=w590) -> ((hi.lo)=w588:u32)
                            n224 = Greater?(x=w588, y=u32 0) -> (0:w586:bool)
                            n225 = Decrement(x=w584) -> (x-1=w585:u16)
                            n226 = Select(t=w585, s=w586, f=w584) -> (s? t:f=w587:u16)
                          }
                          frame 8 {
                            # "RegB=RegB+ RegA(lo)"
                            n227 = Split Number(x=w603) -> (lo(x)=w600:u16)  [unwired: 1 out]
                            n228 = Add(x=w600, y=w599) -> (x+y=w601:u16)
                          }
                          frame 9 {
                            # "RegD<-AI1+par1"
                            n229 = To Word Integer(number=w610) -> (16bit integer=w609:i16)
                            n230 = local read "AI1"() -> (w612:i16)
                            n231 = Add(x=w609, y=w612) -> (x+y=w611:i16)
                          }
                          frame 10 {
                            # "RegD<-RegD*2^par1*par2"
                            n232 = To Word Integer(number=w624) -> (16bit integer=w626:i16)
                            n233 = To Word Integer(number=w625) -> (16bit integer=w627:i16)
                            n234 = Multiply(x=w626, y=w623) -> (x*y=w621:i16)
                            n235 = Scale By Power Of 2(n=w627, x=w621) -> (x*2^n=w622:i16)
                          }
                          frame 11 {
                            # "Sleep counter =par1* memory Block[RegC]"
                            n236 = Greater?(x=w636, y=u32 0) -> (0:w640:bool)
                            n237 = Decrement(x=w638) -> (x-1=w639:u16)
                            n238 = Select(t=w639, s=w640, f=w638) -> (s? t:f=w641:u16)
                          }
                          frame 12 {
                            # "for loop start"
                            # "set fctr to 1"
                            "head ip" <- w647
                          }
                          frame 13 {
                            # "for loop end"
                            n239 = Join Numbers(hi=w657, lo=w656) -> ((hi.lo)=w655:u32)
                            "for N" <- w655
                            n240 = local read "head ip"() -> (w658:u16)
                            n241 = Less Or Equal?(x=w655, y=w664) -> (x <= y?=w660:bool)
                            n242 = Increment(x=w664) -> (x+1=w661:u16)
                            n243 = Select(t=u16 1, s=w660, f=w661) -> (s? t:f=w663:u16)
                            "forctr output" <- w663
                            n244 = Select(t=w659, s=w660, f=w658) -> (s? t:f=w665:u16)
                            "nxt ip output" <- w665
                            "for ctr" <- w664
                            "curr ip" <- w659
                          }
                        }
                      }
                      frame 5 {
                        # "If statement"
                        n245 = case shown="6" w676 {
                          tunnel: [w689 w697 w705 w713 w723 w726 w734] -> w678
                          tunnel: w677 -> [w688 w696 w704 w712 w722 w727 w735]
                          tunnel: w671 -> [w682 _ _ _ _ _ _]
                          tunnel: w675 -> [_ _ w700 w707 _ _ _]
                          tunnel: w674 -> [_ w691 _ w706 _ _ _]
                          tunnel: w673 -> [w683 _ _ _ _ w724 w732]
                          tunnel: w672 -> [w681 w690 w699 _ _ w725 _]
                          tunnel: w670 -> [_ _ _ _ _ _ w739]
                          frame 0, Default {
                            # "The if regA =  [par1,par2]"
                            n246 = Number To Boolean Array(number=w688) -> (Boolean array=w686:bool[])
                            n247 = Join Numbers(hi=w682, lo=w681) -> ((hi.lo)=w680:u32)
                            n248 = Equal?(x=w680, y=w683) -> (x = y?=w684:bool)
                            n249 = Replace Array Subset(array=w686, new element=w684, index=0) -> (w685:bool[])
                            n250 = Boolean Array To Number(Boolean array=w685) -> (number=w689:u8)
                          }
                          frame 1 {
                            # "The if  regB >  par1"
                            n251 = Number To Boolean Array(number=w696) -> (Boolean array=w694:bool[])
                            n252 = Greater?(x=w691, y=w690) -> (0:w692:bool)
                            n253 = Replace Array Subset(array=w694, new element=w692, index=0) -> (w693:bool[])
                            n254 = Boolean Array To Number(Boolean array=w693) -> (number=w697:u8)
                          }
                          frame 2 {
                            # "The if  regC=  par1"
                            n255 = Number To Boolean Array(number=w704) -> (Boolean array=w702:bool[])
                            n256 = Equal?(x=w699, y=w700) -> (x = y?=w698:bool)
                            n257 = Replace Array Subset(array=w702, new element=w698, index=0) -> (w701:bool[])
                            n258 = Boolean Array To Number(Boolean array=w701) -> (number=w705:u8)
                          }
                          frame 3 {
                            # "The if  regB> regC"
                            n259 = Number To Boolean Array(number=w712) -> (Boolean array=w710:bool[])
                            n260 = Greater?(x=w706, y=w707) -> (0:w708:bool)
                            n261 = Replace Array Subset(array=w710, new element=w708, index=0) -> (w709:bool[])
                            n262 = Boolean Array To Number(Boolean array=w709) -> (number=w713:u8)
                          }
                          frame 4 {
                            w718 = 3 ("index")
                            # "external trigger rising edge"
                            n263 = Number To Boolean Array(number=w722) -> (Boolean array=w719:bool[])
                            n264 = local read "exttrigger"() -> (w715:bool)
                            n265 = Index Array(array=w719, index=w718) -> (element=w717:bool)
                            n266 = Not(x=w717) -> (.not. x?=w716:bool)
                            n267 = And(x=w715, y=w716) -> (x .and. y?=w714:bool)
                            n268 = Replace Array Subset(array=w719, new element #1=w714, index #1=0 ("index"), new element #2=w715, index #2=w718) -> (w720:bool[])
                            n269 = Boolean Array To Number(Boolean array=w720) -> (number=w723:u8)
                          }
                          frame 5 {
                            # "The if  regA >  par1"
                            n270 = Number To Boolean Array(number=w727) -> (Boolean array=w730:bool[])
                            n271 = Greater?(x=w724, y=w725) -> (0:w728:bool)
                            n272 = Replace Array Subset(array=w730, new element=w728, index=0) -> (w729:bool[])
                            n273 = Boolean Array To Number(Boolean array=w729) -> (number=w726:u8)
                          }
                          frame 6 {
                            # "The if  regA == memoryBlock(regC)"
                            n274 = Number To Boolean Array(number=w735) -> (Boolean array=w737:bool[])
                            n275 = Equal?(x=w732, y=w739) -> (x = y?=w733:bool)
                            n276 = Replace Array Subset(array=w737, new element=w733, index=0) -> (w736:bool[])
                            n277 = Boolean Array To Number(Boolean array=w736) -> (number=w734:u8)
                          }
                        }
                      }
                      frame 6 {
                        # "condition (flags[0]) goto\nuse par1=par2 for normal goto"
                        n278 = Number To Boolean Array(number=w744) -> (Boolean array=w750:bool[])
                        n279 = Index Array(array=w750, index=0) -> (element=w748:bool)
                        n280 = Select(t=w747, s=w748, f=w746) -> (s? t:f=w745:u16)
                      }
                      frame 7 {
                        w759 = 2 ("index")
                        # "make a Not gate of flag(2)"
                        # "push  to FIFO"
                        n281 = case shown="4" w766 {
                          tunnel: w770 -> [w773 _ _ _]
                          tunnel: w769 -> [_ w774 _ _]
                          tunnel: w768 -> [_ _ w775 _]
                          tunnel: [w773 w774 w775 w776] -> w767
                          frame 0, Default {
                            # "push RegA"
                          }
                          frame 1 {
                            # "push RegB"
                          }
                          frame 2 {
                            # "push RegC"
                          }
                          frame 4 {
                            n282 = local read "AI1"() -> (w776:i16)
                          }
                        }
                        n283 = Number To Boolean Array(number=w760) -> (Boolean array=w764:bool[])
                        n284 = Index Array(array=w764, index=w759) -> (element=w763:bool)
                        n285 = Not(x=w763) -> (.not. x?=w762:bool)
                        n286 = Replace Array Subset(array=w764, new element=w762, index=w759) -> (w765:bool[])
                        n287 = Increment(x=w757) -> (x+1=w756:i16)
                        n288 = Boolean Array To Number(Boolean array=w765) -> (number=w761:u8)
                        n289 = xnode ("FIFO Write")("Element"=w767, "Timeout"=0) -> ()  [unwired: 1 in, 2 out]
                      }
                      frame 8 {
                        # "Stop and reset program"
                        n290 = Number To Boolean Array(number=w783) -> (Boolean array=w786:bool[])
                        n291 = Replace Array Subset(array=w786, new element=TRUE ("new element/subarray"), index=7) -> (w785:bool[])
                        n292 = Boolean Array To Number(Boolean array=w785) -> (number=w784:u8)
                      }
                      frame 9 {
                        # "Cold Lab Specific instructions"
                        n293 = case shown="0, Default" w793 {
                          tunnel: w812 -> [w825 w830 w846]
                          tunnel: w811 -> [w824 w829 w847]
                          tunnel: w810 -> [w821 w831 w844]
                          tunnel: [w821 w831 w844] -> w809
                          tunnel: w808 -> [w820 w832 w843]
                          tunnel: [w820 w832 w843] -> w807
                          tunnel: w806 -> [w819 w833 w842]
                          tunnel: [w819 w833 w842] -> w805
                          tunnel: w804 -> [w818 w834 w841]
                          tunnel: [w818 w834 w841] -> w803
                          tunnel: w802 -> [w817 w835 w840]
                          tunnel: [w817 w835 w840] -> w801
                          tunnel: w800 -> [w816 w836 w839]
                          tunnel: [w816 w836 w839] -> w799
                          tunnel: [w815 w837 w838] -> w798
                          tunnel: w797 -> [w815 w837 w838]
                          tunnel: w796 -> [w814 w828 w845]
                          tunnel: [w814 w828 w845] -> w795
                          tunnel: w794 -> [_ w827 _]
                          tunnel: w793 -> [w813 _ _]
                          tunnel: w792 -> [_ _ w848]
                          frame 0, Default {
                            # "Run Square wave generator"
                            n294 = Greater?(x=w813, y=u8 0) -> (0:w822:bool)
                            n295 = Join Numbers(hi=w825, lo=w824) -> ((hi.lo)=w826:u32)
                            n296 = local write "square wave  on?"(w822) -> ()
                            n297 = local write "square wave period"(w826) -> ()
                          }
                          frame 1 {
                            # "start compression"
                            n298 = Set Occurrence(w827) -> ()
                            n299 = local write "ramp time [10*us]"(w829) -> ()
                            n300 = local write "End Current"(w830) -> ()
                          }
                          frame 2 {
                            n301 = local write "cooling ramp time [10*us]"(w847) -> ()
                            n302 = Set Occurrence(w848) -> ()
                            n303 = local write "End Cooling Intensity"(w846) -> ()
                          }
                        }
                      }
                      frame 10 {
                        n304 = local write "trigger AI1"(TRUE) -> ()
                      }
                    }
                    "control flags" <- w344
                    n305 = Number To Boolean Array(number=w344) -> (Boolean array=w353:bool[])
                    n306 = Index Array(array=w353, index=7) -> (element=w351:bool)
                    n307 = Or(x=w351, y="halt processor") -> (x .or. y?=w350:bool)
                    "IP address" <- w305
                    "ReA" <- w339
                    "RegB" <- w346
                    "RegC" <- w338
                    "FIFO size" <- w319
                    "RegD" <- w318
                  }
                  n308 = node-c288(w302) -> ()
                }
                frame True {
                }
              }
            }
          }
          frame #1 {
            n309 = local write "Run program"(FALSE ("Run program")) -> ()
          }
        }
      }
    }
  }
  n310 = while {
    tunnel: w3 -> [w867]
    stop <- FALSE stop-if-true
    n311 = flat-sequence {
      tunnel: w867 -> [w869]
      frame #0 {
        n312 = Wait on Occurrence(2:w869) -> ()  [unwired: 2 in, 1 out]
      }
      frame #1 {
        n313 = local read "AO5_pigeon"() -> (w870:i16)
        n314 = local write "AO5"(w870) -> ()
      }
    }
  }
  n315 = node-c288() -> (w12:T2)  [unwired: 1 in]
  n316 = while {
    shift-right: [w871] -> _
    shift-left: i16 0 -> [w872]
    stop <- FALSE stop-if-true
    n317 = case shown="False" "analog ramp on" {
      tunnel: [w875 w879] -> w871
      tunnel: w872 -> [w875 w876]
      frame False {
      }
      frame True {
        n318 = local read "analog ramp period"() -> (w878:i16)
        n319 = Less?(x=w876, y=w878) -> (x < y?=w877:bool)
        n320 = Increment(x=w876) -> (x+1=w880:i16)
        n321 = Not(x=w877) -> (.not. x?=w882:bool)
        n322 = Select(t=i16 0, s=w882, f=w880) -> (s? t:f=w879:i16)
        n323 = xnode "FPGA I/O Node"("Connector0/AO7"=w876) -> ()  [unwired: 1 in, 1 out]
        "Numeric" <- w876
      }
    }
  }
  n324 = while {
    stop <- FALSE stop-if-true
    n325 = xnode "FPGA I/O Node"() -> ("Connector0/AI0"=→"Connector0/AI0":i16)  [unwired: 1 in, 1 out]
  }
  n326 = timed-loop {
    shift-right: [w886] -> _
    shift-left: u64 0 -> [w889]
    shift-right: [w888] -> _
    shift-left: TRUE -> [w887]
    timing: w12 -> [_]
    timing-out: [_] -> w11
    tunnel: [w888] -> _
    stop <- _ stop-if-true
    n327 = case shown="False" "square wave  on?" {
      tunnel: w889 -> [w891 w895]
      tunnel: [w890 w899] -> w888
      tunnel: w887 -> [w890 w898]
      tunnel: [w891 w896] -> w886
      frame False {
      }
      frame True {
        n328 = local read "square wave period"() -> (w894:i32)
        n329 = xnode "FPGA I/O Node"("Connector1/DIO6"=w898) -> ()  [unwired: 1 in, 1 out]
        n330 = Less?(x=w895, y=w894) -> (x < y?=w892:bool)
        n331 = Not(x=w892) -> (.not. x?=w893:bool)
        n332 = Increment(x=w895) -> (x+1=w901:u64)
        n333 = Not(x=w898) -> (.not. x?=w900:bool)
        n334 = Select(t=i16 0, s=w893, f=w901) -> (s? t:f=w896:u64)
        n335 = Greater Or Equal?(x=w896, y=w894) -> (x >= y?=w897:bool)
        n336 = Select(t=w900, s=w897, f=w898) -> (s? t:f=w899:bool)
      }
    }
  }
  n337 = node-c288(w11) -> ()
